vi "Build Class Path.vi"(8 "Error In":errorcluster, 10 "Class Name":string="JMETestSolutions.Instrument.lvclass", 11 "Class Relative Path":path) -> (0 "Error Out":errorcluster, 3 "Class Path":path)   [LabVIEW 2020, in "JMETestSolutions.Instrument.lvlib" / "JMETestSolutions.Instrument.lvclass"]
uses:
  JMETestSolutions.Instrument.lvclass
  <vilib>/Utility/LVLibp/NI_PackedLibraryUtility.lvlib
panel:
  out "path":path
  out "dup path":path
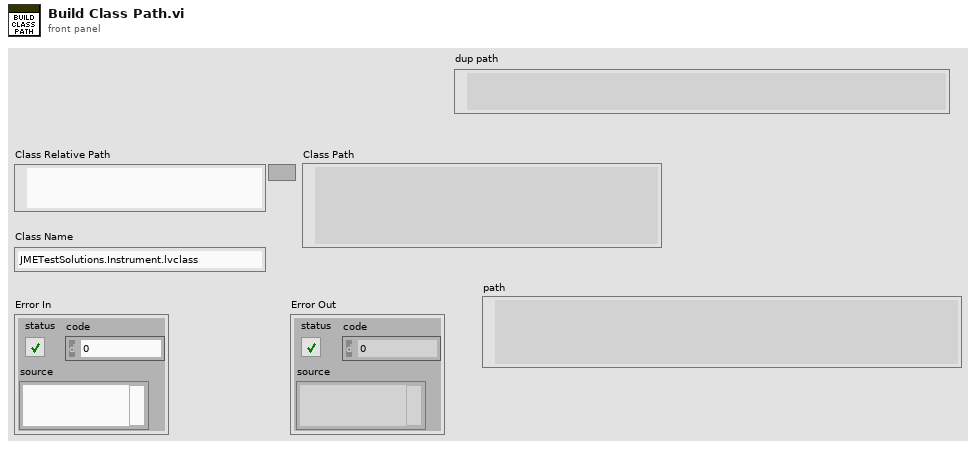
[diagram p1: front panel]
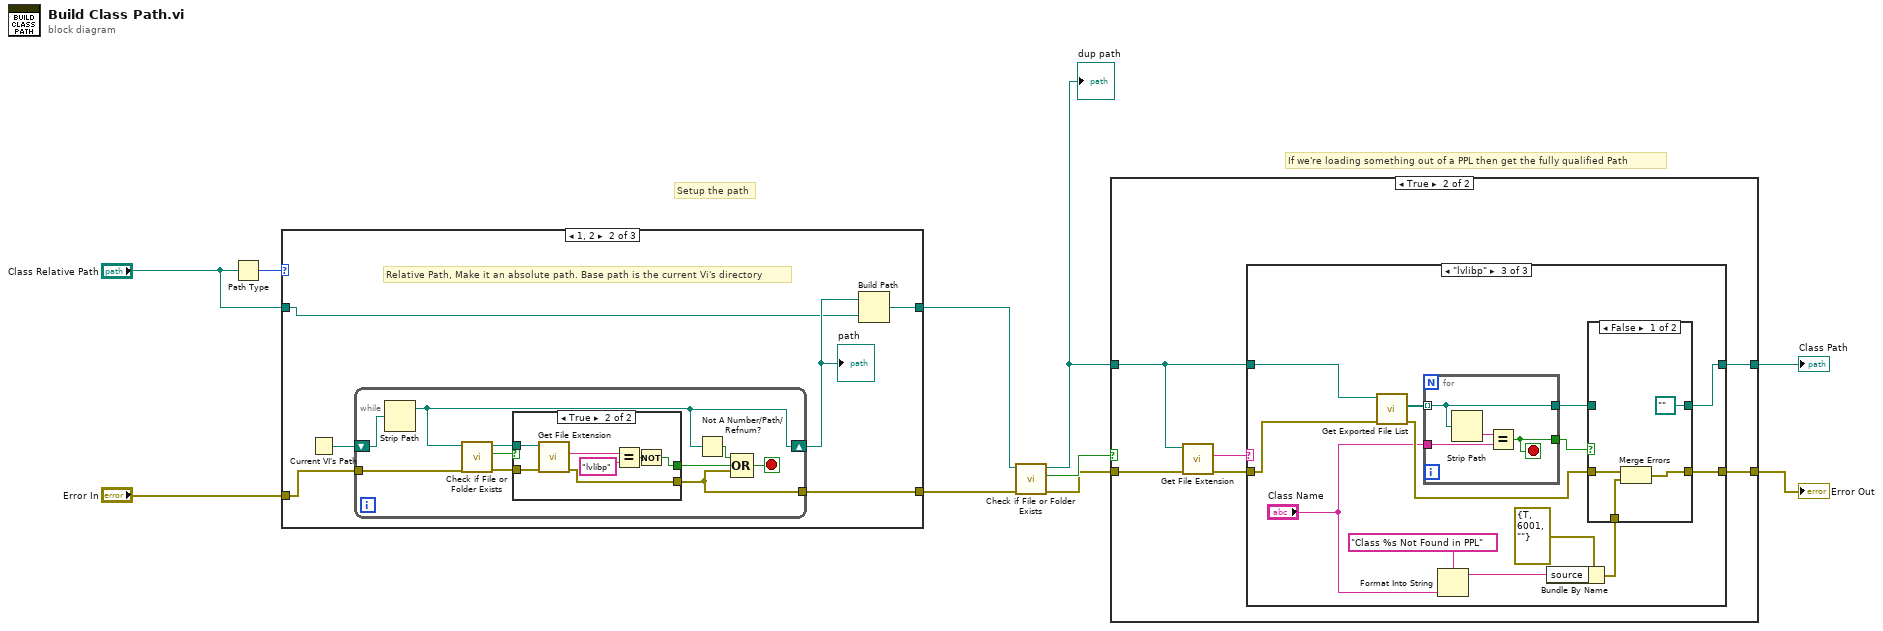
[diagram p0: block diagram]
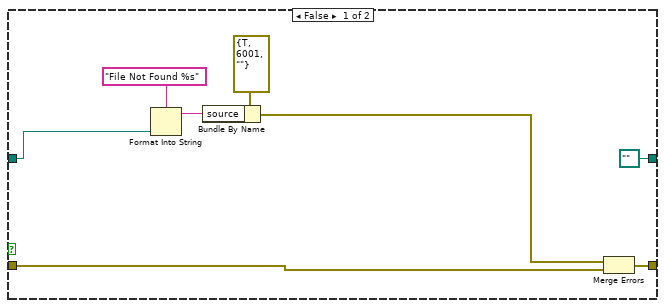
[diagram p2: hidden frame]
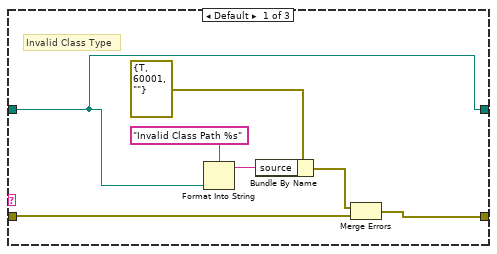
[diagram p3: hidden frame]
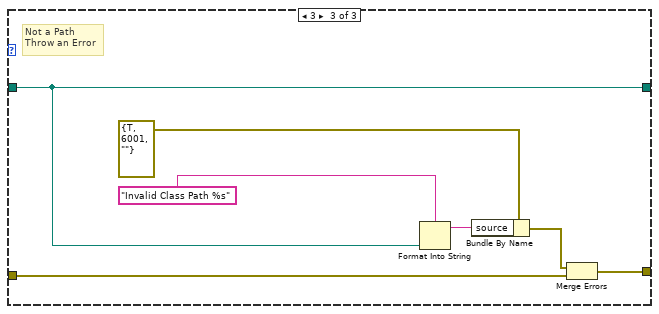
[diagram p8: hidden frame]
diagram:
  # "If we're loading something out of a PPL then get the fully qualified Path"
  # "Setup the path"
  n1 = Path Type(1:"Class Relative Path") -> (0:w10:i16)
  n2 = case shown="1, 2" w10 {
    tunnel: [w12 w17 w43] -> w7
    tunnel: "Class Relative Path" -> [w12 w15 w43]
    tunnel: "Error In" -> [w11 w14 w39]
    tunnel: [w11 w13 w38] -> w8
    frame 0, Default {
      # "Absolute Path\nPass it on"
    }
    frame 1, 2 {
      # "Relative Path, Make it an absolute path. Base path is the current Vi's directory"
      n3 = Current VI's Path() -> (path=w18:path)
      n4 = while {
        shift-right: [w24] -> w16
        shift-left: w18 -> [w26]
        tunnel: w14 -> [w25]
        tunnel: [w19] -> w13
        stop <- w28 stop-if-true
        n5 = Strip Path(path=w26) -> (stripped path=w24:path)  [unwired: 1 out]
        n6 = call <vilib>:"Check if File or Folder Exists.vi"("error in (no error)"=w25, "path"=w24) -> ("error out"=w21:errorcluster, "file or folder exists?"=w22:bool, "dup path"=w23:path)  [unwired: 7 in]
        n7 = case shown="True" w22 {
          selector: w22 -> [w30 _]
          tunnel: w23 -> [_ w37]
          tunnel: w21 -> [w29 w36]
          tunnel: [w30 w32] -> w20
          tunnel: [w29 w35] -> w19
          frame False {
          }
          frame True {
            n8 = call <vilib>:"Get File Extension.vi"("error in (no error)"=w36, "file"=w37) -> ("error out"=w35:errorcluster, "lowercase file extension"=w34:string)  [unwired: 5 in, 3 out]
            n9 = Equal?(x=w34, y="lvlibp") -> (x = y?=w31:bool)
            n10 = Not(x=w31) -> (.not. x?=w32:bool)
          }
        }
        n11 = Not A Number/Path/Refnum?(number/path/refnum=w24) -> (NaN/Path/Refnum?=w27:bool)
        n12 = Compound Arithmetic op=OR(w27, w20, w19) -> (w28:bool)
      }
      "path" <- w16
      n13 = Build Path(base path=w16, name or relative path=w15) -> (appended path=w17:path)
    }
    frame 3 {
      # "Not a Path\nThrow an Error"
      n14 = Format Into String(format string="Invalid Class Path %s", w43) -> (resulting string=w41:string)  [unwired: 2 in, 1 out]
      n15 = Bundle By Name(cluster=errorcluster {"status"=TRUE, "code"=6001, "source"=""} ("Error In"), "source"=w41) -> (w40:errorcluster)
      n16 = Merge Errors(w40, w39) -> (w38:errorcluster)
    }
  }
  n17 = call <vilib>:"Check if File or Folder Exists.vi"("error in (no error)"=w8, "path"=w7) -> ("error out"=w4:errorcluster, "file or folder exists?"=w6:bool, "dup path"=w5:path)  [unwired: 7 in]
  "dup path" <- w5
  n18 = case shown="True" w6 {
    tunnel: w5 -> [w46 w55]
    tunnel: w4 -> [w48 w58]
    tunnel: [w47 w54] -> w2
    tunnel: [path "" ("path") w53] -> w3
    frame False {
      n19 = Format Into String(format string="File Not Found %s", w46) -> (resulting string=w50:string)  [unwired: 2 in, 1 out]
      n20 = Bundle By Name(cluster=errorcluster {"status"=TRUE, "code"=6001, "source"=""} ("Error In"), "source"=w50) -> (w49:errorcluster)
      n21 = Merge Errors(w49, w48) -> (w47:errorcluster)
    }
    frame True {
      n22 = call <vilib>:"Get File Extension.vi"("error in (no error)"=w58, "file"=w55) -> ("error out"=w56:errorcluster, "lowercase file extension"=w57:string)  [unwired: 5 in, 3 out]
      n23 = case shown="\"lvlibp\"" w57 {
        tunnel: w56 -> [w61 w66 w79]
        tunnel: w55 -> [w59 w67 w70]
        tunnel: [w60 w66 w78] -> w54
        tunnel: [w59 w67 w68] -> w53
        frame Default {
          # "Invalid Class Type"
          n24 = Format Into String(format string="Invalid Class Path %s", w59) -> (resulting string=w63:string)  [unwired: 2 in, 1 out]
          n25 = Bundle By Name(cluster=errorcluster {"status"=TRUE, "code"=60001, "source"=""} ("Error In"), "source"=w63) -> (w62:errorcluster)
          n26 = Merge Errors(w62, w61) -> (w60:errorcluster)
        }
        frame "lvclass" {
        }
        frame "lvlibp" {
          n27 = call <vilib>:"Get Exported File List.vi"("error in (no error)"=w79, "packed library path"=w70) -> ("error out"=w77:errorcluster, "paths"=w80:path[])  [unwired: 7 in, 1 out]
          n28 = for {
            tunnel: w80 -> [w87] mode=indexing
            tunnel: "Class Name" -> [w89]
            tunnel: [w88] -> w71
            tunnel: [w87] -> w69
            stop <- w88 stop-if-true
            n29 = Strip Path(path=w87) -> (name=w90:string)  [unwired: 1 out]
            n30 = Equal?(x=w90, y=w89) -> (x = y?=w88:bool)
          }
          n31 = Format Into String(format string="Class %s Not Found in PPL", "Class Name") -> (resulting string=w73:string)  [unwired: 2 in, 1 out]
          n32 = Bundle By Name(cluster=errorcluster {"status"=TRUE, "code"=6001, "source"=""} ("error out"), "source"=w73) -> (w72:errorcluster)
          n33 = case shown="False" w71 {
            tunnel: [w84 w86] -> w78
            tunnel: w77 -> [w83 w86]
            tunnel: w72 -> [w82 _]
            tunnel: w69 -> [_ w85]
            tunnel: [path "" ("path") w85] -> w68
            frame False {
              n34 = Merge Errors(w83, w82) -> (w84:errorcluster)
            }
            frame True {
            }
          }
        }
      }
    }
  }
  "Error Out" <- w2
  "Class Path" <- w3
